vi "correlation.vi"(0 "selection range":cluster{"x0":dbl, "x1":dbl} {"x1" format="%.2f"; "x0" format="%.2f"}, 1 "binning":dbl format="%.2f", 2 "MCS":T2(array[cluster]) {"binning (s)" format="%.2f"; "binning (s)" format="%.2f"}, 3 "rawdata":T3) -> ()   [LabVIEW 2009]
panel:
  out "Selected MCS":u32[](graph)
  out "Busy":bool
  in  "Aceptor Channel":i32
  in  "Calculate":bool
  out "Autocorrelation":cluster{dbl, dbl}[](graph)
  out "Power Spectrum":T1(graph)
  in  "Exit":bool
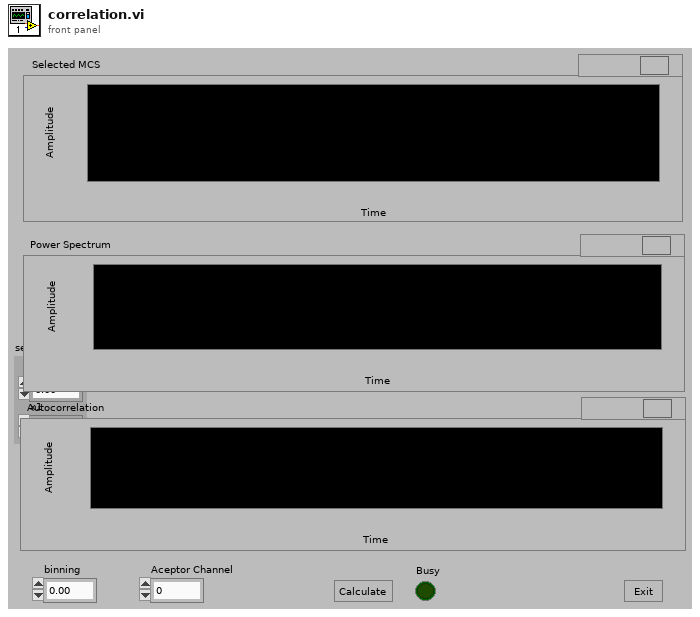
[diagram p1: front panel]
types:
  T1 = cluster{"Power Spectrum FFT {X} Frequency":dbl[], "Power Spectrum FFT {X}":dbl[]}
  T2 = cluster{"binning (s)":dbl, "binning (s)":dbl, "Histogram: h(x)":u32[]}[]
  T3 = cluster{"router channels":u8[], "macro times":u32[], "micro times":u16[], "invalid times":u32[], "gap times":u32[]}
  T4 = cluster{"binning (s)":dbl, "binning (s)":dbl, "Histogram: h(x)":u32[]}
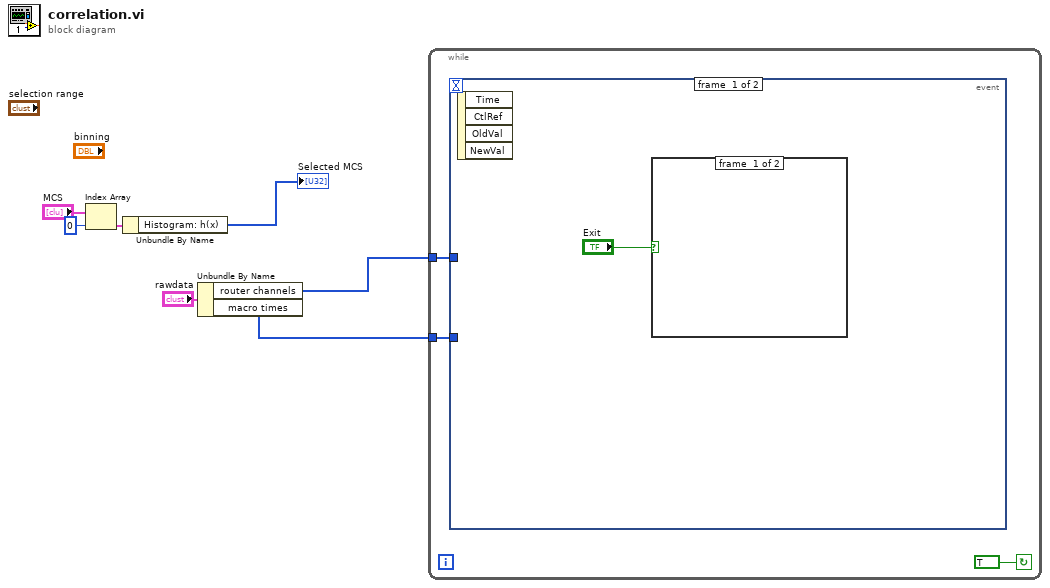
[diagram p0: block diagram]
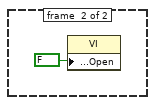
[diagram p2: hidden frame]
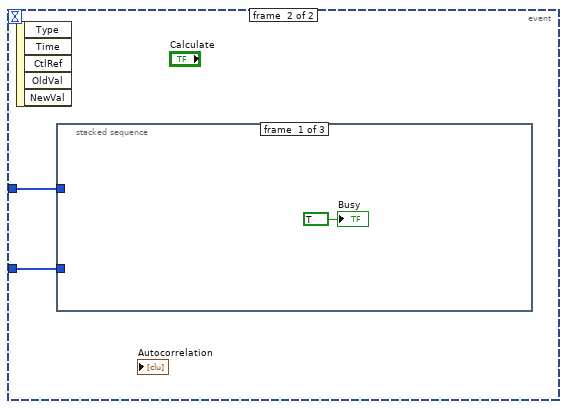
[diagram p3: hidden frame]
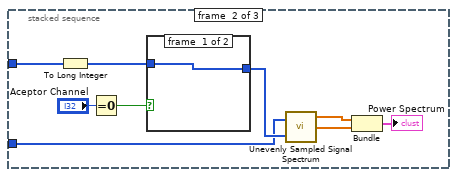
[diagram p4: hidden frame]
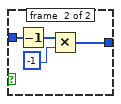
[diagram p5: hidden frame]
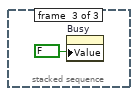
[diagram p6: hidden frame]
diagram:
  n1 = Index Array(array="MCS", index=0) -> (element=w5:T4)
  n2 = Unbundle By Name(w5) -> ("Histogram: h(x)"=→"Selected MCS":u32[])
  n3 = Unbundle By Name("rawdata") -> ("router channels"=w2:u8[], "macro times"=w1:u32[])
  n4 = while {
    tunnel: w2 -> [w9]
    tunnel: w1 -> [w8]
    stop <- TRUE continue-if-true
    n5 = event shown="[1] \"Calculate\": Value Change" {
      selector: _ -> [_ _]
      dyn-events: _ -> [_ _]
      timeout: _ -> [_ _]
      tunnel: w9 -> [_ w14]
      tunnel: w8 -> [_ w13]
      event #0 {
        n6 = event-data() -> ()  [unwired: 1 in, 4 out]
        n7 = case shown="True" "Exit" {
          frame #0 {
          }
          frame #1 {
            n8 = property class="VI"("Front Panel Window:Open"=FALSE) -> ()  [unwired: 2 in, 2 out]
          }
        }
      }
      event #1 {
        n9 = event-data() -> ()  [unwired: 1 in, 5 out]
        n10 = stacked-sequence {
          tunnel: w14 -> [_ w18 _]
          tunnel: w13 -> [_ w16 _]
          frame #0 {
            "Busy" <- TRUE ("Busy")
          }
          frame #1 {
            n11 = To Long Integer(number=w18) -> (32bit integer=w22:i32[])
            n12 = Equal To 0?(x="Aceptor Channel") -> (x = 0?=w23:bool)
            n13 = case shown="False" w23 {
              tunnel: w22 -> [w25 w29]
              tunnel: [w25 w26] -> w17
              frame #0 {
              }
              frame #1 {
                n14 = Decrement(x=w29) -> (x-1=w28:i32[])
                n15 = Multiply(x=w28, y=-1) -> (x*y=w26:i32[])
              }
            }
            n16 = call "Unevenly Sampled Signal Spectrum.vi"("XTime"=w16, "X"=w17) -> ("Power Spectrum FFT {X} Frequency"=w21:dbl[], "Power Spectrum FFT {X}"=w20:dbl[])  [unwired: 1 out]
            n17 = Bundle("Power Spectrum FFT {X} Frequency"=w21, "Power Spectrum FFT {X}"=w20) -> (→"Power Spectrum":T1)  [unwired: 1 in]
          }
          frame #2 {
            n18 = property on="Busy" class="Boolean (strict)"("Value"=FALSE ("Busy")) -> ()  [unwired: 2 in, 2 out]
          }
        }
      }
    }
  }
